vi "Setup.vi"(8 "error in (no error)":errorcluster, 10 "Report Strategy.lvclass":refnum<class "Report Strategy.lvclass">) -> (0 "error out":errorcluster, 3 "Test out":refnum<class "Test.lvclass">)   [LabVIEW 2020, in "Test.lvclass"]
uses:
  Test.lvclass
  Report Strategy/Report Strategy.lvclass
  Test.lvclass/Test.ctl
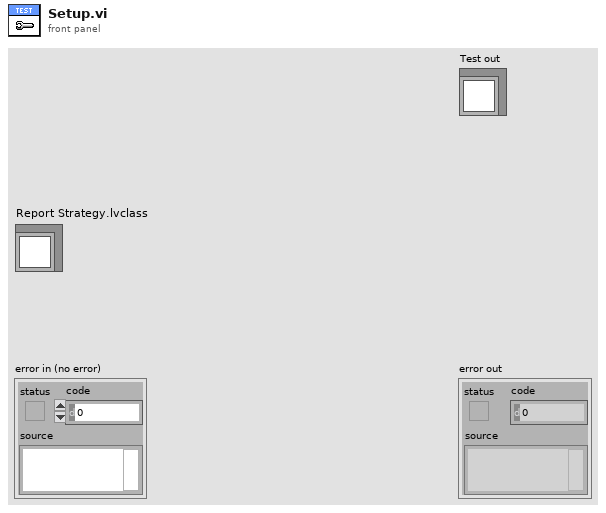
[diagram p1: front panel]
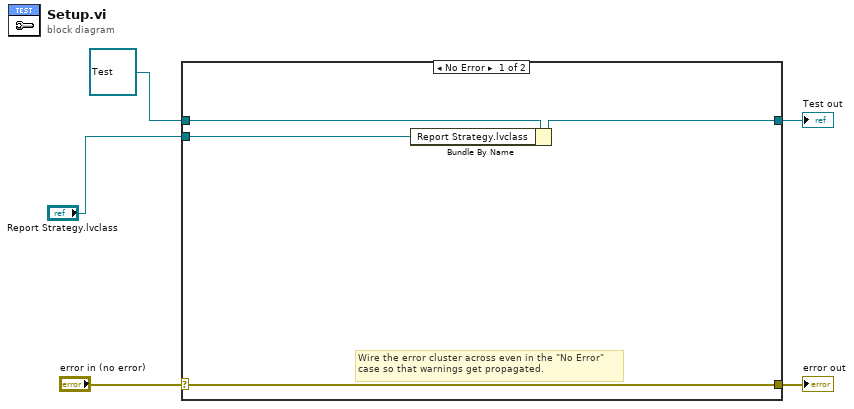
[diagram p0: block diagram]
diagram:
  n1 = case shown="No Error" "error in (no error)" {
    selector: "error in (no error)" -> [w8 w11]
    tunnel: [w8 w11] -> w4
    tunnel: [w7 w10] -> w2
    tunnel: refnum<class "Test.lvclass"> refnum ("Test in") -> [w9 w10]
    tunnel: "Report Strategy.lvclass" -> [w6 _]
    frame No Error {
      # "Wire the error cluster across even in the \"No Error\"\ncase so that warnings get propagated."
      n2 = Bundle By Name(cluster=w9, "Report Strategy.lvclass"=w6) -> (w7:refnum<class "Test.lvclass">)
    }
    frame Error {
    }
  }
  "error out" <- w4
  "Test out" <- w2
